vi "STP Protocol_Init.vi"(0 "object in":refnum<class "STP Protocol.lvclass">, 5 "Init Data":T3={"TxID"=0, "RxID"=0, "CMD"=0, "RQ Data"=[], "+veResponseCode"=160, "ResponseTimeout (S)"=0.1} {"ResponseTimeout (S)" format="%#_13g"; "+veResponseCode" format="%x"; "CMD" items=["TSW_VERSION(130)"=130, "WAIT_EVENT(132)"=132, "SEQUENCER(133)"=133, "TSW_RESET(150)"=150, "CONFIG_ECU(151)"=151, "TEST_CORE (152)"=152, "TEST_WATCHDOG (153)"=153, "TEST_MONITORING (154)"=154, "READ_MEMORY (162)"=162, "WRITE_ERASE_MEMORY (164)"=164, "COMM_EXTERNAL (190)"=190, "COMM_INTERNAL (195)"=195, "GET_ANALOG_INPUT (210)"=210, "GET_DIGITAL_INPUT (211)"=211, "GET_FREQUENCY_INPUT (212)"=212, "TEST_INPUT_STRUCTURE (214)"=214, "GENERATE_OUTPUT_SIGNAL (220)"=220, "GENERATE_SYNCHRONIZED_OUTPUT_SIGNALS (221)"=221, "eDCU_Specific (250)"=250]; "RxID" format="%.0x"; "TxID" format="%.0x"}, 7 "CAN HAL Lib.lvlib:NI-XNET":refnum<class "NI-XNET.lvclass">, 9 "CAN Init Data":T1={"XNET Interface"="", "Baud Rate"=500000, "CAN:Termination"=0, "Echo Transmit?"=FALSE, "scope (normal)"=1} {"scope (normal)" items=["Normal", "Session Only", "Interface Only", "Session Only Blocking"]; "CAN:Termination" items=["Off", "On"]; "Baud Rate" format="%.0p"}, 11 "error in (no error)":errorcluster) -> (4 "object out":refnum<class "STP Protocol.lvclass">, 15 "error out":errorcluster)   [LabVIEW 2023, in "HardwareAbstractionLayer_LVOOP.lvlib" / "CAN Application Protocols Lib.lvlib" / "STP Protocol.lvclass"]
uses:
  STP Protocol.lvclass
  Ctrls/STP Input Data.ctl
  Ctrls/STP CMD.ctl
  CAN Lib/CAN_class/Ctrls/CAN Init Ctrl.ctl
  <vilib>/xnet/xnet.llb/XNET Control Scope.ctl
  CAN Lib/NI-XNET_class/NI-XNET.lvclass
  STP Protocol.lvclass/STP Protocol.ctl
  CAN Lib/CAN_class/CAN.lvclass
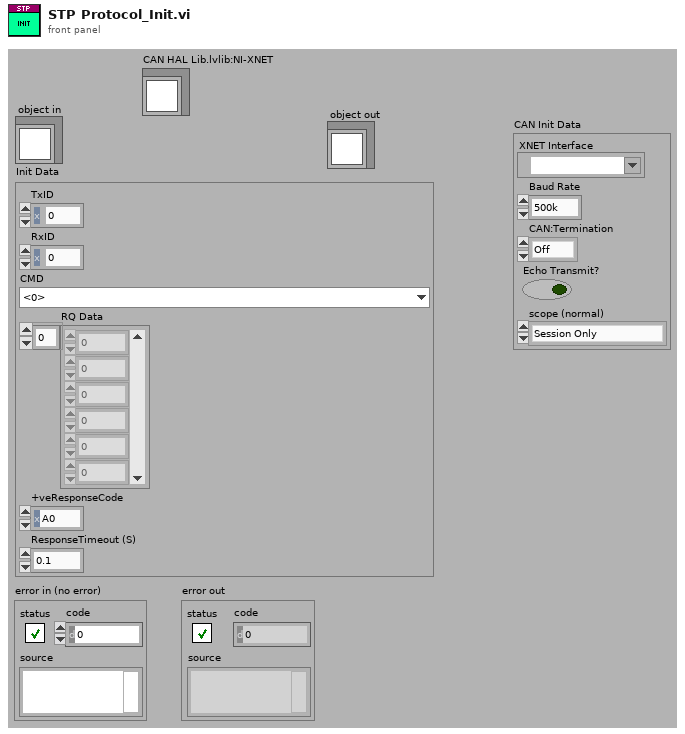
[diagram p1: front panel]
types:
  T1 = typedef "HardwareAbstractionLayer_LVOOP.lvlib/CAN HAL Lib.lvlib/CAN.lvclass/CAN Init Ctrl.ctl" = cluster{"XNET Interface":refnum<k21>, "Baud Rate":u64, "CAN:Termination":u32, "Echo Transmit?":bool, "scope (normal)":T2}
  T2 = typedef "XNET Control Scope.ctl" = u32
  T3 = typedef "HardwareAbstractionLayer_LVOOP.lvlib/CAN Application Protocols Lib.lvlib/STP Protocol.lvclass/STP Input Data.ctl" = cluster{"TxID":u32, "RxID":u32, "CMD":T4, "RQ Data":u8[], "+veResponseCode":u8, "ResponseTimeout (S)":dbl}
  T4 = typedef "HardwareAbstractionLayer_LVOOP.lvlib/CAN Application Protocols Lib.lvlib/STP Protocol.lvclass/STP CMD.ctl" = u8
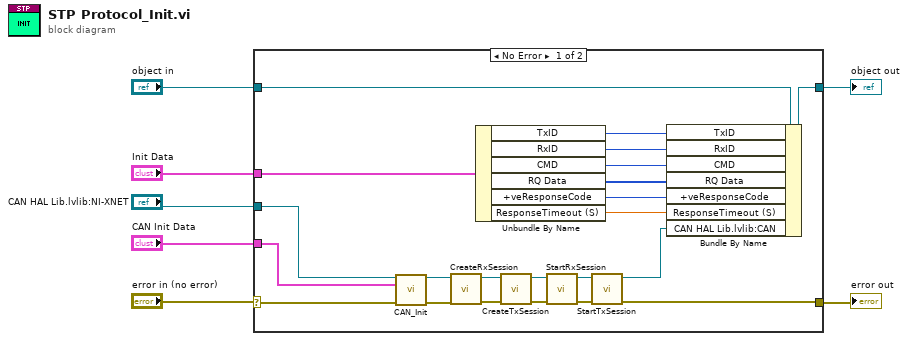
[diagram p0: block diagram]
diagram:
  n1 = case shown="No Error" "error in (no error)" {
    selector: "error in (no error)" -> [w15 w30]
    tunnel: "object in" -> [w29 w31]
    tunnel: [w28 w31] -> w6
    tunnel: [w14 w30] -> w4
    tunnel: "CAN Init Data" -> [w13 _]
    tunnel: "Init Data" -> [w12 _]
    tunnel: "CAN HAL Lib.lvlib:NI-XNET" -> [w11 _]
    frame No Error {
      n2 = call-dynamic "CAN_Init.vi"("object in"=w11, "CAN Init Data"=w13, "error in (no error)"=w15) -> ("object out"=w19:refnum<class "NI-XNET.lvclass">, "error out"=w18:errorcluster)  [unwired: 11 in]
      n3 = call-dynamic "CreateRxSession.vi"("error in (no error)"=w18, "NI-XNET in"=w19) -> ("error out"=w21:errorcluster, "NI-XNET out"=w20:refnum<class "NI-XNET.lvclass">)  [unwired: 8 in]
      n4 = Unbundle By Name(w12) -> ("TxID"=w27:u32, "RxID"=w26:u32, "CMD"=w25:T4, "RQ Data"=w24:u8[], "+veResponseCode"=w10:u8, "ResponseTimeout (S)"=w9:dbl)
      n5 = call-dynamic "CreateTxSession.vi"("error in (no error)"=w21, "NI-XNET in"=w20) -> ("error out"=w16:errorcluster, "NI-XNET out"=w17:refnum<class "NI-XNET.lvclass">)  [unwired: 8 in]
      n6 = call-dynamic "StartRxSession.vi"("error in (no error)"=w16, "NI-XNET in"=w17) -> ("error out"=w23:errorcluster, "NI-XNET out"=w22:refnum<class "NI-XNET.lvclass">)  [unwired: 8 in]
      n7 = call-dynamic "StartTxSession.vi"("error in (no error)"=w23, "NI-XNET in"=w22) -> ("error out"=w14:errorcluster, "NI-XNET out"=w8:refnum<class "NI-XNET.lvclass">)  [unwired: 8 in]
      n8 = Bundle By Name(cluster=w29, "TxID"=w27, "RxID"=w26, "CMD"=w25, "RQ Data"=w24, "+veResponseCode"=w10, "ResponseTimeout (S)"=w9, "CAN HAL Lib.lvlib:CAN"=w8) -> (w28:refnum<class "STP Protocol.lvclass">)
    }
    frame Error {
    }
  }
  "object out" <- w6
  "error out" <- w4
